vi "test Pointer Lifecycle.vi"(8 "error in (no error)":errorcluster, 11 "Test Case in":refnum<class "Lifecycle Tests.lvclass">) -> (0 "error out":errorcluster, 3 "Test Case out":refnum<class "Lifecycle Tests.lvclass">)   [LabVIEW 2017, in "Pointer Tests.lvlib" / "Lifecycle Tests.lvclass"]
uses:
  Lifecycle Tests.lvclass
  Source/Classes/Pointer/Pointer.lvclass
  Source/Classes/Pointer/Public/New/New (1B).vi
  <vilib>/addons/_JKI Toolkits/VI Tester/TestCase.llb/TestCase.lvclass
  C:/Program Files (x86)/National Instruments/LabVIEW 2017/vi.lib/addons/_JKI Toolkits/VI Tester/TestCase.llb/TestCase.lvclass
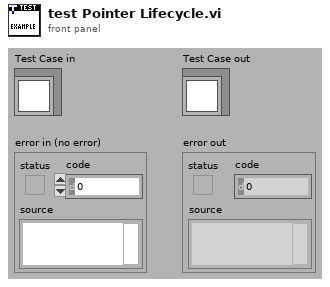
[diagram p1: front panel]
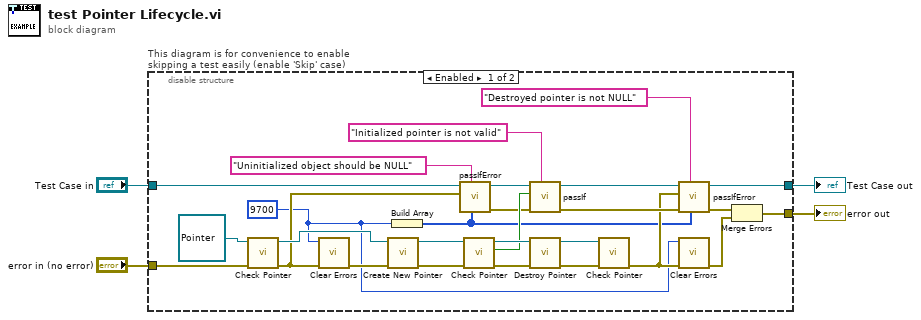
[diagram p0: block diagram]
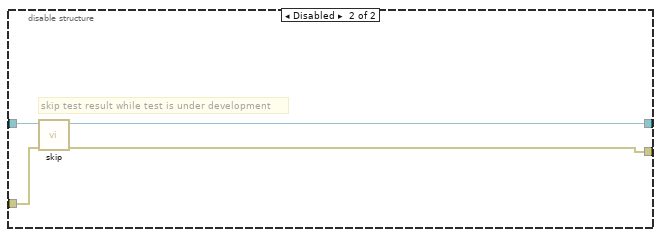
[diagram p2: hidden frame]
diagram:
  n1 = disable-structure "This diagram is for convenience to enable skipping a test easily (enable 'Skip' case)" shown="Enabled" {
    disable-tunnel: "Test Case in" -> [w14 w35]
    disable-tunnel: [w15 w33] -> w2
    disable-tunnel: [w22 w34] -> w1
    disable-tunnel: "error in (no error)" -> [w10 w32]
    frame Enabled {
      w11 = 9700 ("pass error code (0=any error code)")
      n2 = call "Check Pointer.vi"("error in (no error)"=w10, "Pointer in"=refnum<class "Pointer.lvclass"> refnum) -> ("error out"=w18:errorcluster, "Pointer out"=w30:refnum<class "Pointer.lvclass">)  [unwired: 7 in, 1 out]
      n3 = call <vilib>:"Clear Errors.vi"("error in (no error)"=w18, "specific error code to clear (0: all)"=w11) -> ("error out"=w17:errorcluster)  [unwired: 4 in, 1 out]
      n4 = call-poly "Create New Pointer.vi"("error in (no error)"=w17, "Pointer type"=w30) -> ("error out"=w28:errorcluster, "Pointer"=w29:refnum<class "Pointer.lvclass">)  [unwired: 8 in]
      n5 = Build Array(w11) -> (w12:i32[])
      n6 = call-dynamic "passIfError.vi"("passing error codes (default = any error code)"=w12, "custom report message (\"\")"="Uninitialized object should be NULL" ("task (\"\")"), "error"=w18, "TestCase in"=w14) -> ("error out"=w25:errorcluster, "TestCase out"=w13:refnum<class "Lifecycle Tests.lvclass">)  [unwired: 6 in]
      n7 = call "Check Pointer.vi"("error in (no error)"=w28, "Pointer in"=w29) -> ("error out"=w8:errorcluster, "LabVIEW pointer?"=w26:bool, "Pointer out"=w27:refnum<class "Pointer.lvclass">)  [unwired: 7 in]
      n8 = call-dynamic "passIf.vi"("custom report message (\"\")"="Initialized pointer is not valid" ("task (\"\")"), "error in (no error)"=w25, "pass"=w26, "TestCase in"=w13) -> ("error out"=w24:errorcluster, "TestCase out"=w16:refnum<class "Lifecycle Tests.lvclass">)  [unwired: 6 in]
      n9 = call "Destroy Pointer.vi"("error in (no error)"=w8, "Pointer in"=w27) -> ("error out"=w19:errorcluster, "Pointer out"=w20:refnum<class "Pointer.lvclass">)  [unwired: 8 in]
      n10 = call "Check Pointer.vi"("error in (no error)"=w19, "Pointer in"=w20) -> ("error out"=w21:errorcluster)  [unwired: 7 in, 2 out]
      n11 = call-dynamic "passIfError.vi"("passing error codes (default = any error code)"=w12, "custom report message (\"\")"="Destroyed pointer is not NULL" ("task (\"\")"), "error in (no error)"=w24, "error"=w21, "TestCase in"=w16) -> ("error out"=w23:errorcluster, "TestCase out"=w15:refnum<class "Lifecycle Tests.lvclass">)  [unwired: 5 in]
      n12 = call <vilib>:"Clear Errors.vi"("error in (no error)"=w21, "specific error code to clear (0: all)"=w11) -> ("error out"=w9:errorcluster)  [unwired: 4 in, 1 out]
      n13 = Merge Errors(w23, w9) -> (w22:errorcluster)
    }
    frame Disabled {
      # "skip test result while test is under development"
      n14 = call <vilib>:"skip.vi"("error in (no error)"=w32, "TestCase in"=w35) -> ("error out"=w34:errorcluster, "TestCase out"=w33:refnum<class "Lifecycle Tests.lvclass">)  [unwired: 8 in]
    }
  }
  "error out" <- w1
  "Test Case out" <- w2
